vi "Create Client Context.vi"(8 "error in (no error)":errorcluster) -> (0 "error out":errorcluster, 3 "ContextID out":T1)   [LabVIEW 2019, in "grpc-lvsupport.lvlib"]
uses:
  grpc-lvsupport.lvlib
  Shared/grpcId.ctl
  <vilib>/Utility/error.llb/Error Cluster From Error Code.vi
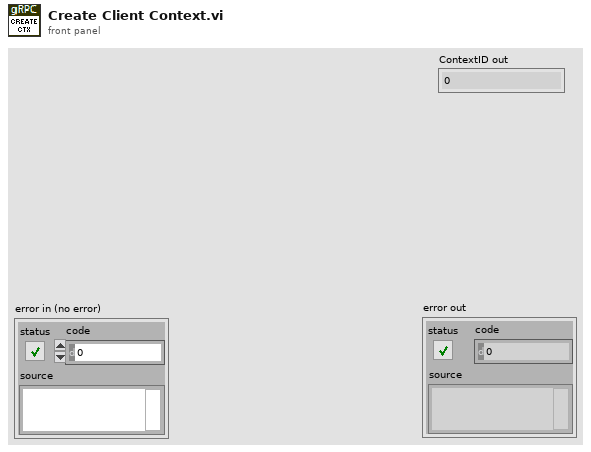
[diagram p1: front panel]
types:
  T1 = typedef "grpc-lvsupport.lvlib/grpcId.ctl" = u64
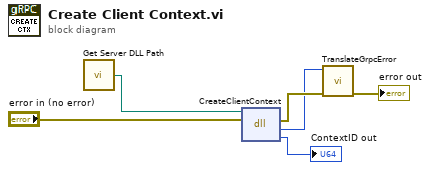
[diagram p0: block diagram]
diagram:
  n1 = call "Get Server DLL Path.vi"() -> ("Server dll path"=w6:path)
  n2 = dll-call lib="?" fn="CreateClientContext"(path in=w6, error in="error in (no error)") -> (error out=w3:errorcluster, "return type"=w2:i32, "contextId"=→"ContextID out":u64)  [unwired: 2 in, 1 out]
  n3 = call "TranslateGrpcError.vi"("error in"=w3, "Error Code"=w2) -> ("error out"=→"error out":errorcluster)  [unwired: 9 in]
